vi "ABB Test No Load.vi"() -> ()   [LabVIEW 2017]
uses:
  Temp error msg.ctl
  <vilib>/Analysis/baseanly.llb/Mean (DBL).vi
  ABB global.vi
  <vilib>/Analysis/NI_AALPro.lvlib
  <vilib>/Analysis/NI_AALBase.lvlib
panel:
  in  "Temp error":T1="Error: Temperature measurement "
  in  "Case Constant\n(See Context Help)":i32
  in  "Additional Mech Loss (kW)":dbl
  in  "show fit":bool
  out "Additional Temperatures  (°C)":string[][](table)
  in  "Simulate volts":dbl(slide) max=1800.0
  out "Temperatures  (°C)":string[][](table)
  out "Losses (kW)":string[][](table)
  out "Auto Readings":cluster{"%":dbl[], "Recorded":bool[]}
  out "In Range?":bool[](array[boolean])
  out "saved Readings":dbl[][](array[numeric])
  out "% rated voltage":dbl format="%.1f"
  out "Rated Volts":dbl
  out "Serial number":string
  out "W.O number":string
  out "Power":string[][](table)
  out "Voltage":string[][](table)
  out "Current":string[][](table)
  out "Norma 5000 Error":string
  in  "Record":bool
  out "Readings":string[][](table)
  in  "View":enum16{"Graph", "Readings"}(ring)
  out "Number readings":i32
  out "Status":enum16{"Stopped", "Running"}(ring)
  out "Timedate":string
  in  "End test":bool
  in  "Start":bool
  in  "Read Mode":enum16{"Auto", "Manual"}(ring)
  in  "Exit":bool
  out "Separation of losses":cluster{dbl[], "Best Linear Fit":dbl[]}[](graph)
  # "No Load Test"
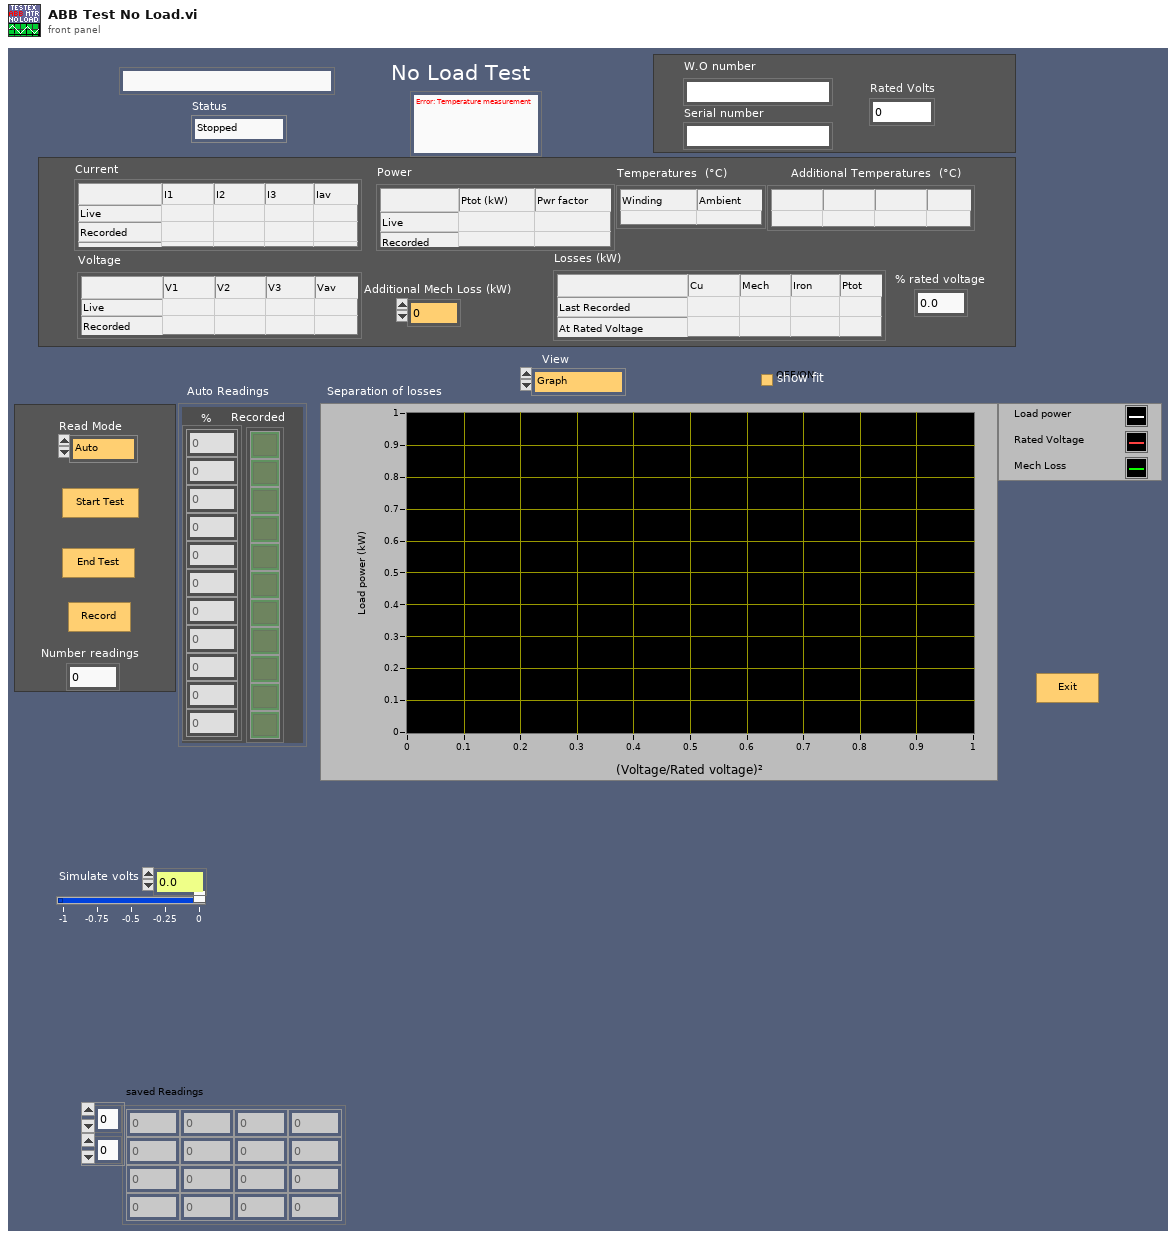
[diagram p1: front panel]
types:
  T1 = typedef "Temp error msg.ctl" = string
  T2 = cluster{"Voltage":dbl, "Current":dbl, "Power":dbl, "power factor":dbl}
  T3 = cluster{"VT Primary":dbl, "VT Secondary":dbl, "CT  Primary":dbl, "CT Secondary":dbl, "Current Shunt":enum16{"Internal", "External"}, "Avg interval":dbl}
  T4 = cluster{"VT Primary":dbl, "VT Secondary":dbl, "CT  Primary":dbl, "CT Secondary":dbl, "Current Shunt":enum16{"Internal", "External"}, "Averaging interval (secs)":dbl}
  T5 = cluster{"Visa sesssion":refnum<visa-resource-name>, "error":errorcluster}
  T6 = cluster{"Simulate Norma":bool, "Norma 5000 Address":u8, "WebDaq IP Address":string, "Simulate cDAQ":bool}
  T7 = cluster{"Number Values":i32, "Tolerance ":dbl, "Value (ratio)":dbl[], "Hold time (sec)":dbl}
  T8 = cluster{"temp. alloc":i32[], "category":i32[], "Category names":string[], "Category none names":string[]}
  T9 = cluster{"PCu":dbl, "Pmech":dbl, "PFe":dbl, "Ptot":dbl, "Ambient":dbl, "I1":dbl, "I2":dbl, "I3":dbl, "Wdg Temp":dbl}
  T10 = cluster{"V":dbl, "A":dbl, "W":dbl, "VA":dbl, "VAr":dbl, "Pf":dbl}
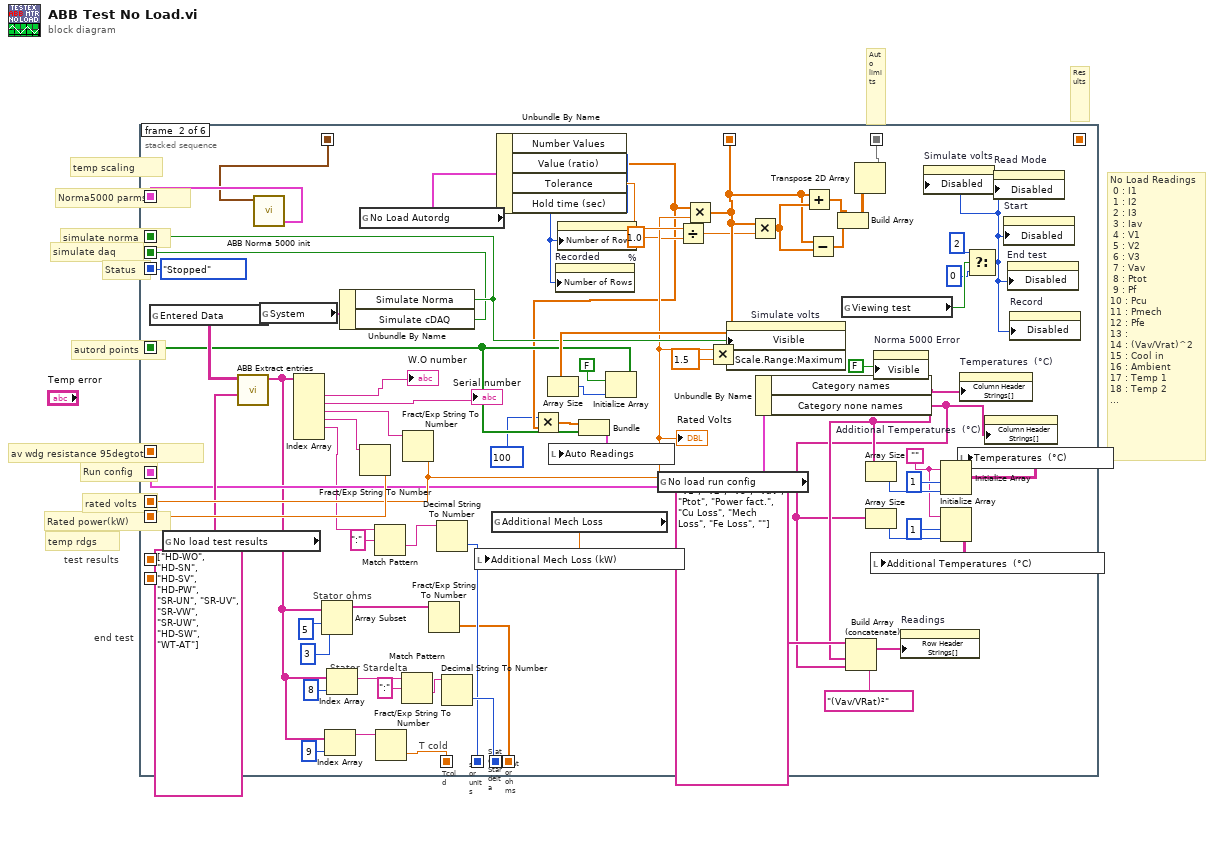
[diagram p0: block diagram]
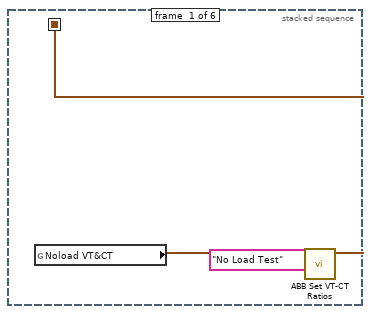
[diagram p2: hidden frame]
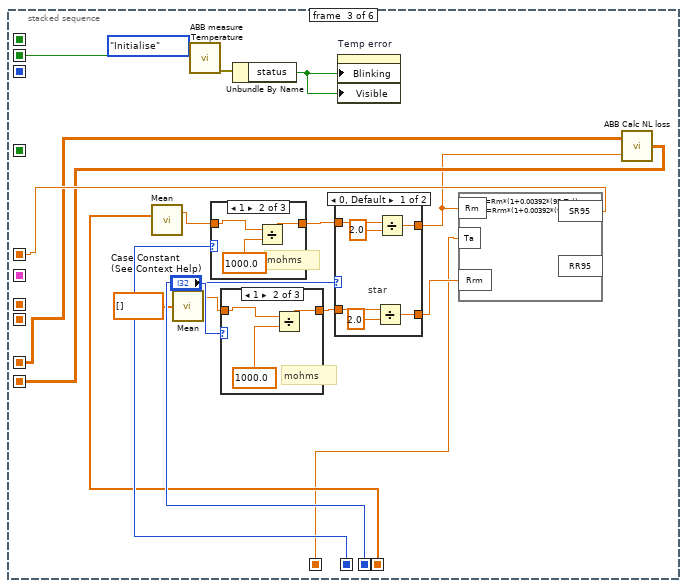
[diagram p3: hidden frame]
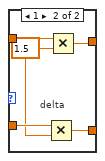
[diagram p4: hidden frame]
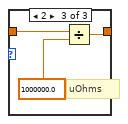
[diagram p6: hidden frame]
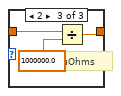
[diagram p8: hidden frame]
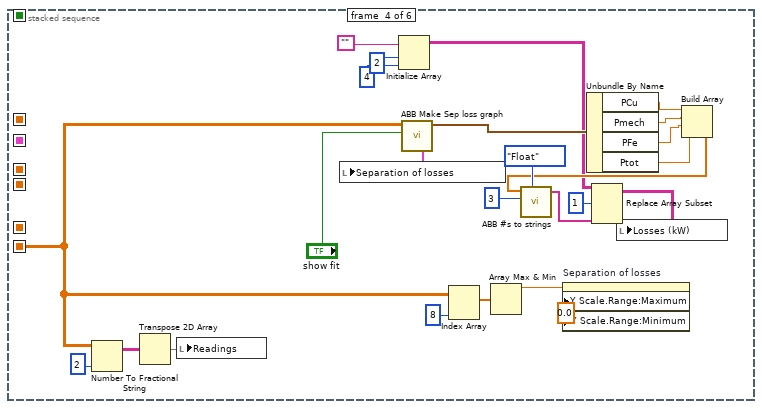
[diagram p9: hidden frame]
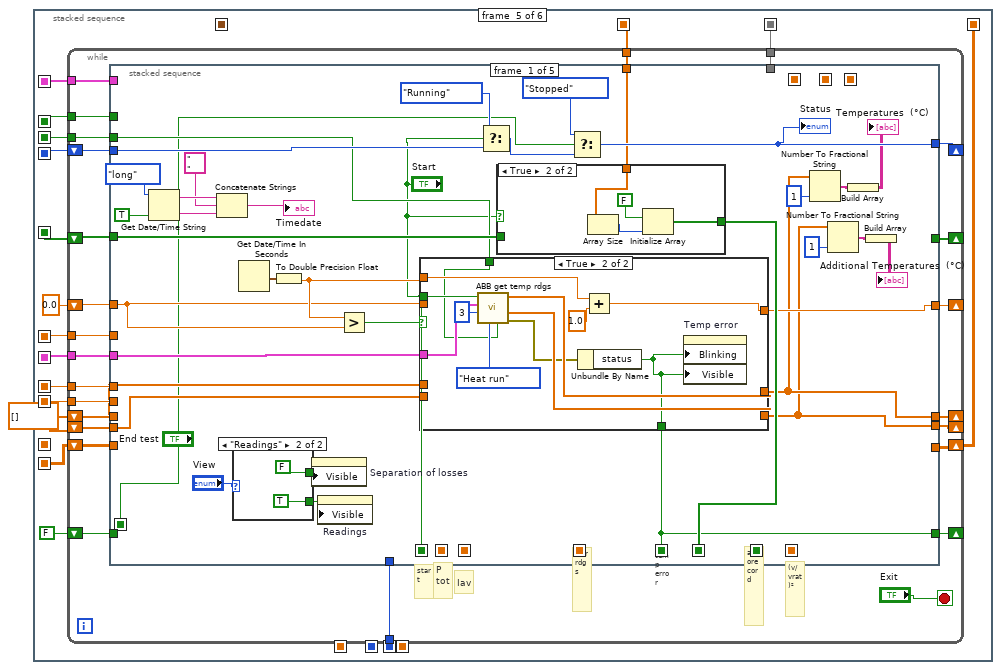
[diagram p10: hidden frame]
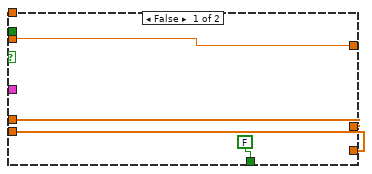
[diagram p11: hidden frame]
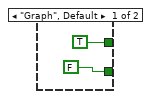
[diagram p13: hidden frame]
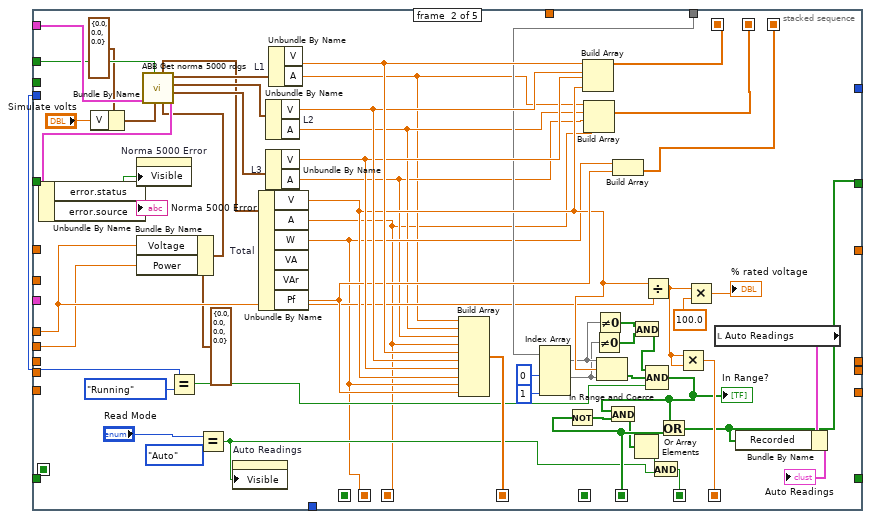
[diagram p14: hidden frame]
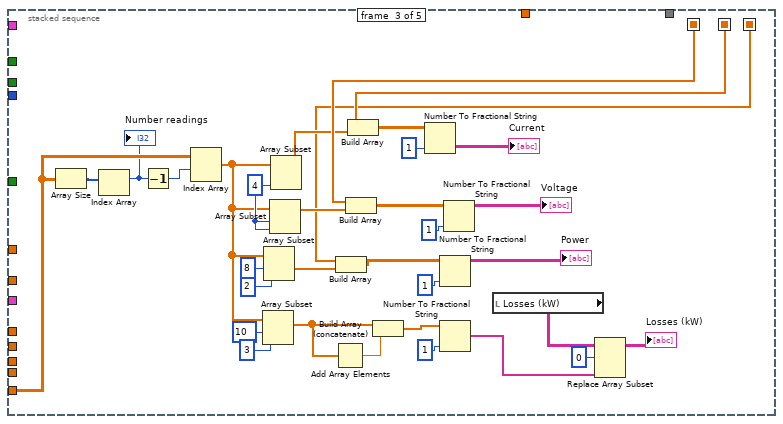
[diagram p15: hidden frame]
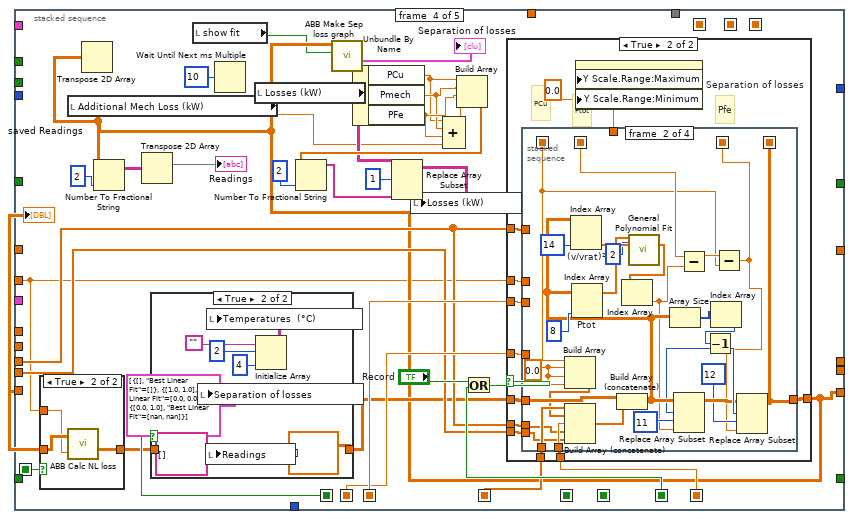
[diagram p16: hidden frame]
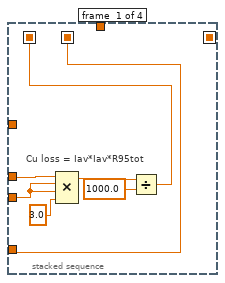
[diagram p20: hidden frame]
diagram:
  # "end test"
  # "test results"
  # "stator ohms"
  # "stator units"
  # "Tcold"
  # "Stator Stardelta"
  # "No Load Readings\n 0 : I1\n 1 : I2\n 2 : I3\n 3 : Iav\n 4 : V1\n 5 : V2\n 6 : V3\n 7 : Vav\n 8 : Ptot\n 9 : Pf\n10 : Pcu\n11 : Pmech\n12 : Pfe\n13 :\n14 : (Vav/Vrat)^2\n15 : Cool in\n16 : Ambient\n17 : Temp 1\n18 : Temp 2\n..."
  # "simulate daq"
  # "temp scaling"
  # "Results"
  # "temp rdgs"
  # "Run config"
  # "Rated power(kW)"
  # "autord points"
  # "Auto limits"
  # "av wdg resistance 95degtot"
  # "rated volts"
  # "simulate norma"
  # "Norma5000 parms"
  # "Status"
  n1 = stacked-sequence {
    seq-local: [_ enum16{"Stopped", "Running"}."Stopped" ("Status") _ _ _ _] -> [_ _ _ _ w160 _]
    seq-local: [_ w73 _ _ _ _] -> [_ _ _ _ w159 w458]
    seq-local: [_ w59 _ _ _ _] -> [_ _ _ _ w158 w457]
    seq-local: [_ w58 _ _ _ _] -> [_ _ _ _ w157 _]
    seq-local: [_ w46 _ _ _ _] -> [_ _ w81 _ _ _]
    seq-local: [_ _ w82 _ _ _] -> [_ _ _ _ w156 _]
    seq-local: [_ w24 _ _ _ _] -> [_ _ _ _ w155 _]
    seq-local: [_ w65 _ _ _ _] -> [_ _ _ _ w153 _]
    seq-local: [_ w63 _ _ _ _] -> [_ _ _ _ w154 _]
    seq-local: [_ w60 _ _ _ _] -> [_ _ _ _ w152 _]
    seq-local: [_ w26 _ _ _ _] -> [_ _ _ _ w150 _]
    seq-local: [_ _ _ _ w149 _] -> [_ _ _ _ _ w455]
    seq-local: [_ w37 _ _ _ _] -> [_ _ w78 _ w148 w452]
    seq-local: [_ w15 _ _ _ _] -> [_ _ w86 _ w146 _]
    seq-local: [w1 _ _ _ _ _] -> [_ w11 _ _ _ w454]
    seq-local: [_ w10 _ _ _ _] -> [_ _ w83 _ _ _]
    seq-local: [_ w9 _ _ _ _] -> [_ _ w87 _ _ _]
    seq-local: [_ w8 _ _ _ _] -> [_ _ w85 _ _ _]
    seq-local: [_ _ w80 _ _ _] -> [_ _ _ w120 w145 _]
    frame #0 {
      n2 = global read "ABB global.vi" "Noload VT&CT"() -> (w3:T3)
      n3 = call "ABB Set VT-CT Ratios.vi"("Test name"="No Load Test", "VT and CT Ratios"=w3) -> ("VT and CT Ratios out"=w1:T4)  [unwired: 9 in]
    }
    frame #1 {
      w28 = ""
      # "T cold"
      # "Stator Stardelta"
      # "Stator ohms"
      n4 = global read "ABB global.vi" "Entered Data"() -> (w55:string[][])
      n5 = global read "ABB global.vi" "No load test results"() -> (w46:dbl[][])
      n6 = call "ABB Extract entries.vi"("Entry IDs"=string[] ["HD-WO", "HD-SN", "HD-SV", "HD-PW", "SR-UN", "SR-UV", "SR-VW", "SR-UW", "HD-SW", "WT-AT"], "Entry table in"=w55) -> ("Selected Entries"=w13:string[])  [unwired: 9 in]
      n7 = call "ABB Norma 5000 init.vi"("VT and CT Ratios"=w11) -> ("norma 5000 parms out"=w73:T5)  [unwired: 10 in]
      n8 = global read "ABB global.vi" "System"() -> (w72:T6)
      n9 = Index Array(array=w13) -> (element #1=→"W.O number":string, element #2=→"Serial number":string, element #3=w52:string, element #4=w51:string, element #5=w6:string)  [unwired: 6 in, 1 out]
      n10 = Array Subset(array=w13, index=5, length=3) -> (w48:string[])
      n11 = Index Array(array=w13, index=9) -> (element=w12:string)
      n12 = Index Array(array=w13, index=8) -> (element=w18:string)
      n13 = Unbundle By Name(w72) -> ("Simulate Norma"=w59:bool, "Simulate cDAQ"=w37:bool)
      n14 = global read "ABB global.vi" "No Load Autordg"() -> (w62:T7)
      n15 = Fract/Exp String To Number(string=w51) -> (number=w60:dbl)  [unwired: 3 in, 1 out]
      n16 = Match Pattern(string=w6, regular expression=":") -> (after substring=w5:string)  [unwired: 1 in, 3 out]
      n17 = Fract/Exp String To Number(string=w12) -> (number=w10:dbl)  [unwired: 3 in, 1 out]
      n18 = Match Pattern(string=w18, regular expression=":") -> (after substring=w16:string)  [unwired: 1 in, 3 out]
      n19 = Fract/Exp String To Number(string=w52) -> (number=w58:dbl)  [unwired: 3 in, 1 out]
      "Rated Volts" <- w58
      n20 = Fract/Exp String To Number(string=w48) -> (number=w8:dbl[])  [unwired: 3 in, 1 out]
      n21 = Decimal String To Number(string=w5) -> (number=w9:i32)  [unwired: 2 in, 1 out]
      n22 = Decimal String To Number(string=w16) -> (number=w15:i32)  [unwired: 2 in, 1 out]
      n23 = global read "ABB global.vi" "Additional Mech Loss"() -> (w4:dbl)
      n24 = local write "Additional Mech Loss (kW)"(w4) -> ()
      n25 = Unbundle By Name(w62) -> ("Number Values"=w25:i32, "Value (ratio)"=w23:dbl[], "Tolerance"=w61:dbl)  [unwired: 1 out]
      n26 = Multiply(x=100 ("Numeric"), y=w23) -> (x*y=w21:dbl[])
      n27 = property on="Recorded" class="Arr (strict)"("Number of Rows"=w25) -> ()  [unwired: 2 in, 2 out]
      n28 = property on="%" class="Arr (strict)"("Number of Rows"=w25) -> ()  [unwired: 2 in, 2 out]
      n29 = global read "ABB global.vi" "No load run config"() -> (w26:T8)
      n30 = Divide(x=w61, y=1.0) -> (x/y=w45:dbl)
      n31 = Multiply(x=w23, y=w58) -> (x*y=w63:dbl[])
      n32 = Array Size(array=w63) -> (size(s)=w70:i32)
      n33 = Initialize Array(FALSE, w70) -> (w24:bool[])
      n34 = Bundle(w21, w24) -> (w22:cluster{dbl[], bool[]})  [unwired: 1 in]
      n35 = local write "Auto Readings"(w22) -> ()
      n36 = Multiply(x=w58, y=1.5) -> (x*y=w56:dbl)
      n37 = property on="Simulate volts" class="Slide (strict)"("Visible"=w59, "Scale.Range:Maximum"=w56) -> ()  [unwired: 2 in, 2 out]
      n38 = Multiply(x=w63, y=w45) -> (x*y=w67:dbl[])
      n39 = Unbundle By Name(w26) -> ("Category names"=w33:string[], "Category none names"=w30:string[])
      n40 = Add(x=w63, y=w67) -> (x+y=w68:dbl[])
      n41 = Subtract(x=w63, y=w67) -> (x-y=w64:dbl[])
      n42 = Build Array(w68, w64) -> (w66:dbl[][])
      n43 = global read "ABB global.vi" "Viewing test"() -> (w41:bool)
      n44 = Build Array (concatenate)(string[] ["I1", "I2", "I3", "Iav", "V1", "V2", "V3", "Vav", "Ptot", "Power fact.", "Cu Loss", "Mech Loss", "Fe Loss", ""], "(Vav/VRat)²", w33, w30) -> (w42:string[])
      n45 = Transpose 2D Array(2D array=w66) -> (transposed array=w65:dbl[][])
      n46 = Array Size(array=w33) -> (size(s)=w35:i32)
      n47 = Array Size(array=w30) -> (size(s)=w27:i32)
      n48 = property on="Norma 5000 Error" class="Str"("Visible"=FALSE) -> ()  [unwired: 2 in, 2 out]
      n49 = property on="Readings" class="Tbl (strict)"("Row Header Strings[]"=w42) -> ()  [unwired: 2 in, 2 out]
      n50 = Initialize Array(w28, 1 ("dimension size"), w35) -> (w32:string[][])
      n51 = Initialize Array(w28, 1 ("dimension size"), w27) -> (w29:string[][])
      n52 = local write "Additional Temperatures  (°C)"(w29) -> ()
      n53 = local write "Temperatures  (°C)"(w32) -> ()
      n54 = property on="Temperatures  (°C)" class="Tbl (strict)"("Column Header Strings[]"=w33) -> ()  [unwired: 2 in, 2 out]
      n55 = Select(t=2, s=w41, f=0) -> (s? t:f=w38:i32)
      n56 = property on="Simulate volts" class="Slide (strict)"("Disabled"=w38) -> ()  [unwired: 2 in, 2 out]
      n57 = property on="Additional Temperatures  (°C)" class="Tbl (strict)"("Column Header Strings[]"=w30) -> ()  [unwired: 2 in, 2 out]
      n58 = property on="Read Mode" class="Enum (strict)"("Disabled"=w38) -> ()  [unwired: 2 in, 2 out]
      n59 = property on="Start" class="Bool"("Disabled"=w38) -> ()  [unwired: 2 in, 2 out]
      n60 = property on="End test" class="Bool"("Disabled"=w38) -> ()  [unwired: 2 in, 2 out]
      n61 = property on="Record" class="Bool"("Disabled"=w38) -> ()  [unwired: 2 in, 2 out]
    }
    frame #2 {
      n62 = call-poly <vilib>:"Mean.vi"("X"=w85) -> ("mean"=w93:dbl)  [unwired: 1 out]
      n63 = call-poly <vilib>:"Mean.vi"("X"=dbl[] []) -> ("mean"=w91:dbl)  [unwired: 1 out]
      n64 = call "ABB measure Temperature.vi"("Simulate"=w78, "Mode"=enum16{"Initialise", "Read", "Close"}."Initialise") -> ("error out"=w76:errorcluster)  [unwired: 7 in, 2 out]
      n65 = case shown="1" w87 {
        tunnel: w93 -> [w112 w115 w118]
        tunnel: [w112 w113 w116] -> w90
        frame 0, Default {
          # "ohms"
        }
        frame 1 {
          # "mohms"
          n66 = Divide(x=w115, y=1000.0) -> (x/y=w113:dbl)
        }
        frame 2 {
          # "uOhms"
          n67 = Divide(x=w118, y=1000000.0) -> (x/y=w116:dbl)
        }
      }
      n68 = case shown="1" "Case Constant\n(See Context Help)" {
        tunnel: w91 -> [w105 w108 w111]
        tunnel: [w105 w106 w109] -> w89
        frame 0, Default {
          # "ohms"
        }
        frame 1 {
          # "mohms"
          n69 = Divide(x=w108, y=1000.0) -> (x/y=w106:dbl)
        }
        frame 2 {
          # "uOhms"
          n70 = Divide(x=w111, y=1000000.0) -> (x/y=w109:dbl)
        }
      }
      n71 = Unbundle By Name(w76) -> ("status"=w75:bool)
      n72 = case shown="0, Default" w86 {
        tunnel: w90 -> [w99 w104]
        tunnel: [w97 w103] -> w79
        tunnel: w89 -> [w96 w102]
        tunnel: [w95 w101] -> w88
        frame 0, Default {
          # "star"
          n73 = Divide(x=w96, y=2.0) -> (x/y=w95:dbl)
          n74 = Divide(x=w99, y=2.0) -> (x/y=w97:dbl)
        }
        frame 1 {
          w100 = 1.5 ("y")
          # "delta"
          n75 = Multiply(x=w102, y=w100) -> (x*y=w101:dbl)
          n76 = Multiply(x=w104, y=w100) -> (x*y=w103:dbl)
        }
      }
      n77 = property on="Temp error" class="Str (strict)"("Blinking"=w75, "Visible"=w75) -> ()  [unwired: 2 in, 2 out]
      n78 = formula code="SR95=Rm*(1+0.00392*(95-Ta));\nRR95=Rrm*(1+0.00392*(95-Ta));"("Rm"=w79, "Ta"=w83, "Rrm"=w88) -> ("SR95"=w82:dbl)  [unwired: 1 out]
      n79 = call "ABB Calc NL loss.vi"("SR95"=w79, "No load test results 2"=w81) -> ("No load test results"=w80:dbl[][])
    }
    frame #3 {
      n80 = Number To Fractional String(number=w120, precision (6)=i16 2) -> (F-format string=w142:string[][])  [unwired: 2 in]
      n81 = Transpose 2D Array(2D array=w142) -> (transposed array=w141:string[][])
      n82 = local write "Readings"(w141) -> ()
      n83 = Initialize Array("", 2, 4) -> (w125:string[][])
      n84 = call "ABB Make Sep loss graph.vi"("Show fit"="show fit", "Results"=w120) -> ("Sep Loss Graph"=w140:cluster{dbl[], dbl[]}[], "Rated V Readings"=w127:T9)  [unwired: 7 in, 1 out]
      n85 = local write "Separation of losses"(w140) -> ()
      n86 = Index Array(array=w120, index (col)=8 ("disabled index (col)")) -> (element=w123:dbl[])  [unwired: 1 in]
      n87 = Array Max & Min(array=w123) -> (max value=w122:dbl)  [unwired: 3 out]
      n88 = property on="Separation of losses" class="XYGraph (strict)"("Y Scale.Range:Maximum"=w122, "Y Scale.Range:Minimum"=0.0) -> ()  [unwired: 2 in, 2 out]
      n89 = Unbundle By Name(w127) -> ("PCu"=w136:dbl, "Pmech"=w135:dbl, "PFe"=w134:dbl, "Ptot"=w133:dbl)
      n90 = Build Array(w136, w135, w134, w133) -> (w126:dbl[])
      n91 = call "ABB #s to strings.vi"("# type"=enum16{"Float", "Relative time HH:MM"}."Float", "Precision"=3, "Numbers in"=w126) -> ("Strings out"=w128:string[])  [unwired: 8 in]
      n92 = Replace Array Subset(array=w125, new element=w128, index (row)=1) -> (w130:string[][])  [unwired: 1 in]
      n93 = local write "Losses (kW)"(w130) -> ()
    }
    frame #4 {
      w147 = dbl[] []
      n94 = while {
        shift-right: [w183] -> _
        shift-left: w160 -> [w184]
        tunnel: w159 -> [w182]
        tunnel: w158 -> [w181]
        tunnel: w157 -> [w180]
        shift-right: [w178] -> w149
        shift-left: w145 -> [w179]
        tunnel: w156 -> [w177]
        shift-right: [w176] -> _
        shift-left: w155 -> [w175]
        tunnel: w154 -> [w174]
        tunnel: w153 -> [w173]
        tunnel: w152 -> [w172]
        shift-right: [w170] -> _
        shift-left: 0.0 -> [w171]
        tunnel: w150 -> [w169]
        shift-right: [w168] -> _
        shift-left: w147 -> [w167]
        tunnel: w148 -> [w166]
        shift-right: [w164] -> _
        shift-left: w147 -> [w165]
        tunnel: w146 -> [w163]
        shift-right: [w162] -> _
        shift-left: FALSE ("status") -> [w161]
        stop <- "Exit" stop-if-true
        # "temp error"
        # "P tot"
        # "Iav"
        # "autorecord"
        # "(v/vrat)²"
        # "pwr rdgs"
        # "start"
        n95 = stacked-sequence {
          seq-local: ["Start" _ _ _ _] -> [_ _ _ w372 _]
          seq-local: [_ w290 _ _ _] -> [_ _ _ w367 _]
          seq-local: [_ w288 _ _ _] -> [_ _ _ w366 _]
          seq-local: [w206 _ _ _ _] -> [_ w283 _ _ _]
          seq-local: [_ w278 _ _ _] -> [_ _ _ w369 _]
          seq-local: [_ w274 _ _ _] -> [_ _ w331 _ _]
          seq-local: [_ w273 _ _ _] -> [_ _ w327 _ _]
          seq-local: [_ w272 _ _ _] -> [_ _ w319 _ _]
          seq-local: [_ w248 _ _ _] -> [_ _ _ w365 _]
          seq-local: [_ w257 _ _ _] -> [_ _ _ w364 _]
          seq-local: ["End test" _ _ _ _] -> [_ _ _ w342 _]
          seq-local: [w186 _ _ _ _] -> [_ _ _ _ w445]
          tunnel: w184 -> [w216 w260 _ _ _]
          tunnel: [w212 _ _ _ _] -> w183
          tunnel: w182 -> [_ w305 _ _ _]
          tunnel: w181 -> [_ w297 _ _ _]
          tunnel: w180 -> [_ w271 _ _ _]
          tunnel: w179 -> [_ _ w337 w343 _]
          tunnel: [_ _ _ w345 _] -> w178
          tunnel: w177 -> [_ _ _ w341 _]
          tunnel: [_ w253 _ _ _] -> w176
          tunnel: w175 -> [w208 _ _ _ _]
          tunnel: w174 -> [w207 _ _ _ _]
          tunnel: w173 -> [_ w286 _ _ _]
          tunnel: w172 -> [_ w255 _ _ _]
          tunnel: w171 -> [w201 _ _ _ _]
          tunnel: [w202 _ _ _ _] -> w170
          tunnel: w169 -> [w200 _ _ _ _]
          tunnel: [w195 _ _ _ _] -> w168
          tunnel: w167 -> [w199 _ _ w363 _]
          tunnel: w166 -> [w198 _ _ _ w442]
          tunnel: w165 -> [w197 _ _ w362 _]
          tunnel: [w189 _ _ _ _] -> w164
          tunnel: w163 -> [_ _ _ _ _]
          tunnel: [w186 _ _ _ _] -> w162
          tunnel: w161 -> [_ _ _ _ w444]
          frame #0 {
            n96 = Get Date/Time String(date format (0)=enum16{"short", "long", "abbreviated"}."long", want seconds? (F)=TRUE) -> (date string=w220:string, time string=w219:string)  [unwired: 1 in]
            n97 = Concatenate Strings(w220, "   ", w219) -> (→"Timedate":string)
            n98 = case shown="\"Readings\"" "View" {
              tunnel: [TRUE FALSE] -> w210
              tunnel: [FALSE TRUE] -> w209
              frame "Graph", Default {
              }
              frame "Readings" {
              }
            }
            n99 = Get Date/Time In Seconds() -> (seconds since 1Jan1904=w204:timestamp)
            n100 = To Double Precision Float(number=w204) -> (double precision float=w203:dbl)
            n101 = property on="Separation of losses" class="XYGraph (strict)"("Visible"=w210) -> ()  [unwired: 2 in, 2 out]
            n102 = property on="Readings" class="Tbl (strict)"("Visible"=w209) -> ()  [unwired: 2 in, 2 out]
            n103 = Greater?(x=w203, y=w201) -> (0:w205:bool)
            n104 = case shown="True" w205 {
              tunnel: w203 -> [_ w238]
              tunnel: [w226 w236] -> w202
              tunnel: w201 -> [w226 _]
              tunnel: w198 -> [_ w229]
              tunnel: w200 -> [_ w235]
              tunnel: [w225 w234] -> w195
              tunnel: w199 -> [w225 _]
              tunnel: w197 -> [w224 _]
              tunnel: [w224 w233] -> w189
              tunnel: "Start" -> [_ w232]
              tunnel: [FALSE ("status") w227] -> w186
              frame False {
              }
              frame True {
                n105 = call "ABB get temp rdgs.vi"("Sim daq"=w229, "sim type"=enum16{"Heat run", "Bearing run"}."Heat run", "# categories"=3, "run config"=w235, "start"=w232) -> ("error out"=w228:errorcluster, "Category none rdgs"=w233:dbl[], "Category rdgs"=w234:dbl[])  [unwired: 3 in, 1 out]
                n106 = Unbundle By Name(w228) -> ("status"=w227:bool)
                n107 = Add(x=w238, y=1.0) -> (x+y=w236:dbl)
                n108 = property on="Temp error" class="Str (strict)"("Blinking"=w227, "Visible"=w227) -> ()  [unwired: 2 in, 2 out]
              }
            }
            n109 = Select(t=enum16{"Stopped", "Running"}."Running", s="Start", f=w216) -> (s? t:f=w214:enum16{"Stopped", "Running"})
            n110 = case shown="True" "Start" {
              tunnel: w207 -> [_ w243]
              tunnel: [w239 w240] -> w206
              tunnel: w208 -> [w239 _]
              frame False {
              }
              frame True {
                n111 = Array Size(array=w243) -> (size(s)=w242:i32)
                n112 = Initialize Array(FALSE, w242) -> (w240:bool[])
              }
            }
            n113 = Select(t=enum16{"Stopped", "Running"}."Stopped", s="End test", f=w214) -> (s? t:f=w212:enum16{"Stopped", "Running"})
            "Status" <- w212
            n114 = Number To Fractional String(number=w195, precision (6)=i16 1) -> (F-format string=w193:string[])  [unwired: 2 in]
            n115 = Number To Fractional String(number=w189, precision (6)=i16 1) -> (F-format string=w191:string[])  [unwired: 2 in]
            n116 = Build Array(w193) -> (→"Temperatures  (°C)":string[][])
            n117 = Build Array(w191) -> (→"Additional Temperatures  (°C)":string[][])
          }
          frame #1 {
            n118 = Bundle By Name(cluster=cluster{"V":dbl, "A":dbl, "pwr factor":dbl} {"V"=0.0, "A"=0.0, "pwr factor"=0.0} ("Simulation rdgs"), "V"="Simulate volts") -> (w267:cluster{"V":dbl, "A":dbl, "pwr factor":dbl})
            n119 = Bundle By Name(cluster=T2 {"Voltage"=0.0, "Current"=0.0, "Power"=0.0, "power factor"=0.0} ("Rated"), "Voltage"=w271, "Power"=w255) -> (w270:T2)
            n120 = call "ABB Get norma 5000 rdgs.vi"("Rated"=w270, "Simulation rdgs"=w267, "simulate"=w297, "norma 5000 parms in"=w305) -> ("norma 5000 parms out"=w299:T5, "L 3"=w300:T10, "L 2"=w301:T10, "L1"=w302:T10, "Total"=w298:T10)  [unwired: 3 in]
            n121 = Unbundle By Name(w299) -> ("error.status"=w304:bool, "error.source"=→"Norma 5000 Error":string)
            n122 = property on="Norma 5000 Error" class="Str"("Visible"=w304) -> ()  [unwired: 2 in, 2 out]
            n123 = Equal?(x=w260, y=enum16{"Stopped", "Running"}."Running") -> (x = y?=w258:bool)
            n124 = Equal?(x="Read Mode", y=enum16{"Auto", "Manual"}."Auto") -> (x = y?=w275:bool)
            n125 = property on="Auto Readings" class="Clust (strict)"("Visible"=w275) -> ()  [unwired: 2 in, 2 out]
            n126 = Unbundle By Name "Total"(w298) -> ("V"=w287:dbl, "A"=w248:dbl, "W"=w257:dbl, "Pf"=w291:dbl)  [unwired: 2 out]
            n127 = Unbundle By Name "L2"(w301) -> ("V"=w293:dbl, "A"=w251:dbl)
            n128 = Unbundle By Name "L3"(w300) -> ("V"=w292:dbl, "A"=w250:dbl)
            n129 = Unbundle By Name "L1"(w302) -> ("V"=w294:dbl, "A"=w249:dbl)
            n130 = Build Array(w249, w251, w250, w248, w294, w293, w292, w287, w257, w291) -> (w290:dbl[])
            n131 = Index Array(array=w286, index (col) #1=0 ("disabled index (col)"), index (col) #2=1 ("index (col)")) -> (element #1=w266:dbl[], element #2=w265:dbl[])  [unwired: 2 in]
            n132 = Not(x=w283) -> (.not. x?=w281:bool[])
            n133 = Build Array(w294, w293, w292, w287) -> (w274:dbl[])
            n134 = Build Array(w249, w251, w250, w248) -> (w273:dbl[])
            n135 = Not Equal To 0?(x=w265) -> (x != 0?=w263:bool[])
            n136 = Not Equal To 0?(x=w266) -> (x != 0?=w264:bool[])
            n137 = In Range and Coerce(upper limit=w266, x=w287, lower limit=w265) -> (In Range?=w282:bool[])  [unwired: 1 out]
            n138 = Build Array(w257, w291) -> (w272:dbl[])
            n139 = And(x=w264, y=w263) -> (x .and. y?=w261:bool[])
            n140 = Divide(x=w287, y=w271) -> (x/y=w289:dbl)
            n141 = Compound Arithmetic op=AND(w261, w282, w258) -> (w262:bool[])
            "In Range?" <- w262
            n142 = And(x=w262, y=w281) -> (x .and. y?=w280:bool[])
            n143 = Or Array Elements(Boolean array=w280) -> (logical OR=w279:bool)
            n144 = And(x=w279, y=w275) -> (x .and. y?=w278:bool)
            n145 = Or(x=w262, y=w283) -> (x .or. y?=w253:bool[])
            n146 = Multiply(x=w289, y=w289) -> (x*y=w288:dbl)
            n147 = Multiply(x=w289, y=100.0) -> (x*y=→"% rated voltage":dbl)
            n148 = local read "Auto Readings"() -> (w254:cluster{"%":dbl[], "Recorded":bool[]})
            n149 = Bundle By Name(cluster=w254, "Recorded"=w253) -> (→"Auto Readings":cluster{"%":dbl[], "Recorded":bool[]})
          }
          frame #2 {
            w334 = 4 ("length")
            n150 = Array Size(array=w337) -> (size(s)=w338:i32[])
            n151 = Index Array(array=w338) -> (element=w313:i32)  [unwired: 1 in]
            "Number readings" <- w313
            n152 = Decrement(x=w313) -> (x-1=w336:i32)
            n153 = Index Array(array=w337, index (row)=w336) -> (element=w316:dbl[])  [unwired: 1 in]
            n154 = Array Subset(array=w316, index=10, length=3) -> (w308:dbl[])
            n155 = Array Subset(array=w316, index=8, length=2) -> (w320:dbl[])
            n156 = Array Subset(array=w316, index=w334, length=w334) -> (w333:dbl[])
            n157 = Array Subset(array=w316, length=w334) -> (w326:dbl[])  [unwired: 1 in]
            n158 = Add Array Elements(numeric array=w308) -> (sum=w306:dbl)
            n159 = Build Array(w319, w320) -> (w321:dbl[][])
            n160 = Build Array(w331, w333) -> (w332:dbl[][])
            n161 = Build Array(w327, w326) -> (w325:dbl[][])
            n162 = Build Array (concatenate)(w308, w306) -> (w307:dbl[])
            n163 = Number To Fractional String(number=w325, precision (6)=i16 1) -> (F-format string=→"Current":string[][])  [unwired: 2 in]
            n164 = Number To Fractional String(number=w321, precision (6)=i16 1) -> (F-format string=→"Power":string[][])  [unwired: 2 in]
            n165 = Number To Fractional String(number=w307, precision (6)=i16 1) -> (F-format string=w309:string[])  [unwired: 2 in]
            n166 = Number To Fractional String(number=w332, precision (6)=i16 1) -> (F-format string=→"Voltage":string[][])  [unwired: 2 in]
            n167 = local read "Losses (kW)"() -> (w312:string[][])
            n168 = Replace Array Subset(array=w312, new element=w309, index (row)=0) -> (→"Losses (kW)":string[][])  [unwired: 1 in]
          }
          frame #3 {
            n169 = case shown="True" w342 {
              tunnel: [w373 w375] -> w344
              tunnel: w343 -> [w373 w376]
              tunnel: w341 -> [_ w374]
              frame False {
              }
              frame True {
                n170 = call "ABB Calc NL loss.vi"("SR95"=w374, "No load test results 2"=w376) -> ("No load test results"=w375:dbl[][])
              }
            }
            n171 = local read "Additional Mech Loss (kW)"() -> (w339:dbl)
            n172 = case shown="True" w372 {
              tunnel: w344 -> [w377 _]
              tunnel: [w377 dbl[][] []] -> w361
              frame False {
              }
              frame True {
                n173 = local write "Separation of losses"(cluster{dbl[], "Best Linear Fit":dbl[]}[] [{[], "Best Linear Fit"=[]}, {[1.0, 1.0], "Best Linear Fit"=[0.0, 0.0]}, {[0.0, 1.0], "Best Linear Fit"=[nan, nan]}] ("Separation of losses")) -> ()
                n174 = local write "Readings"(string[][] [] ("Readings")) -> ()
                n175 = Initialize Array("", 2 ("dimension size"), 4 ("dimension size")) -> (w378:string[][])
                n176 = local write "Temperatures  (°C)"(w378) -> ()
              }
            }
            n177 = local read "show fit"() -> (w340:bool)
            n178 = Wait Until Next ms Multiple(millisecond multiple=u32 10) -> ()  [unwired: 1 out]
            n179 = local read "Losses (kW)"() -> (w351:string[][])
            n180 = Or(x="Record", y=w369) -> (x .or. y?=w370:bool)
            n181 = case shown="True" w370 {
              tunnel: w361 -> [w385 w397]
              tunnel: [w385 w396] -> w345
              tunnel: w367 -> [_ w395]
              tunnel: w363 -> [_ w394]
              tunnel: w366 -> [_ w393]
              tunnel: w341 -> [_ w392]
              tunnel: w365 -> [_ w391]
              tunnel: w363 -> [_ w390]
              tunnel: w364 -> [_ w389]
              tunnel: w362 -> [_ w386]
              frame False {
              }
              frame True {
                # "Pfe"
                # "Ptot"
                # "PCu"
                n182 = stacked-sequence {
                  seq-local: [w401 _ _ _] -> [_ w409 _ _]
                  seq-local: [w399 _ _ _] -> [_ w423 _ _]
                  seq-local: [_ w411 _ _] -> [_ _ _ _]
                  seq-local: [_ w415 _ _] -> [_ _ w439 _]
                  tunnel: w397 -> [_ w431 _ _]
                  tunnel: [_ w415 _ _] -> w396
                  tunnel: w395 -> [_ w429 _ _]
                  tunnel: w394 -> [_ w413 w433 _]
                  tunnel: w393 -> [_ w414 _ _]
                  tunnel: w392 -> [w404 _ _ _]
                  tunnel: w391 -> [w403 _ _ _]
                  tunnel: w390 -> [_ _ _ _]
                  tunnel: w389 -> [w399 _ _ _]
                  tunnel: [_ _ w438 _] -> w387
                  tunnel: w386 -> [_ w412 _ _]
                  frame #0 {
                    # "Cu loss = Iav*Iav*R95tot"
                    n183 = Compound Arithmetic op=MULTIPLY(w404, w403, w403, 3.0 ("value")) -> (w402:dbl)
                    n184 = Divide(x=w402, y=1000.0) -> (x/y=w401:dbl)
                  }
                  frame #1 {
                    w408 = 0.0 ("element")
                    n185 = Build Array(w409, w408, w408, w408) -> (w427:dbl[])
                    n186 = Build Array (concatenate)(w429, w427, w414, w413, w412) -> (w430:dbl[])
                    n187 = Build Array (concatenate)(w431, w430) -> (w422:dbl[][])
                    n188 = Index Array "(v/vrat)²"(array=w422, index (col)=14 ("disabled index (col)")) -> (element=w424:dbl[])  [unwired: 1 in]
                    n189 = Index Array "Ptot"(array=w422, index (col)=8 ("disabled index (col)")) -> (element=w425:dbl[])  [unwired: 1 in]
                    n190 = call <vilib>:"General Polynomial Fit.vi"("Y"=w425, "polynomial order"=2, "X"=w424) -> ("Polynomial Coefficients"=w406:dbl[])  [unwired: 9 in, 3 out]
                    n191 = Index Array(array=w406) -> (element=w405:dbl)  [unwired: 1 in]
                    n192 = Array Size(array=w422) -> (size(s)=w421:i32[])
                    n193 = Subtract(x=w423, y=w405) -> (x-y=w410:dbl)
                    n194 = Index Array(array=w421) -> (element=w420:i32)  [unwired: 1 in]
                    n195 = Decrement(x=w420) -> (x-1=w419:i32)
                    n196 = Replace Array Subset(array=w422, new element=w405, index (row)=w419, index (col)=11) -> (w418:dbl[][])
                    n197 = Subtract(x=w410, y=w409) -> (x-y=w411:dbl)
                    n198 = Replace Array Subset(array=w418, new element=w411, index (row)=w419, index (col)=12) -> (w415:dbl[][])
                  }
                  frame #2 {
                    n199 = Index Array(array=w439, index (col)=8 ("disabled index (col)")) -> (element=w440:dbl[])  [unwired: 1 in]
                    n200 = Number To Fractional String(number=w433, precision (6)=i16 1) -> (F-format string=w434:string[])  [unwired: 2 in]
                    n201 = Array Max & Min(array=w440) -> (max value=w438:dbl)  [unwired: 3 out]
                    n202 = local read "Temperatures  (°C)"() -> (w437:string[][])
                    n203 = Replace Array Subset(array=w437, new element=w434, index (row)=1) -> (w436:string[][])  [unwired: 1 in]
                    n204 = local write "Temperatures  (°C)"(w436) -> ()
                  }
                  frame #3 {
                  }
                }
                n205 = property on="Separation of losses" class="XYGraph (strict)"("Y Scale.Range:Maximum"=w387, "Y Scale.Range:Minimum"=0.0) -> ()  [unwired: 2 in, 2 out]
              }
            }
            n206 = Transpose 2D Array(2D array=w345) -> ()  [unwired: 1 out]
            n207 = Number To Fractional String(number=w345, precision (6)=i16 2) -> (F-format string=w348:string[][])  [unwired: 2 in]
            n208 = Transpose 2D Array(2D array=w348) -> (transposed array=→"Readings":string[][])
            n209 = call "ABB Make Sep loss graph.vi"("Show fit"=w340, "Results"=w345) -> ("Sep Loss Graph"=→"Separation of losses":cluster{dbl[], dbl[]}[], "Rated V Readings"=w350:T9)  [unwired: 7 in, 1 out]
            n210 = Unbundle By Name(w350) -> ("PCu"=w355:dbl, "Pmech"=w356:dbl, "PFe"=w357:dbl)
            n211 = Compound Arithmetic op=ADD(w355, w356, w357, w339) -> (w358:dbl)
            n212 = Build Array(w355, w356, w357, w358) -> (w359:dbl[])
            n213 = Number To Fractional String(number=w359, precision (6)=2 ("Precision")) -> (F-format string=w354:string[])  [unwired: 2 in]
            n214 = Replace Array Subset(array=w351, new element=w354, index (row)=1) -> (w352:string[][])  [unwired: 1 in]
            n215 = local write "Losses (kW)"(w352) -> ()
            "saved Readings" <- w343
          }
          frame #4 {
            n216 = Not(x=w444) -> (.not. x?=w443:bool)
            n217 = And(x=w443, y=w445) -> (x .and. y?=w446:bool)
            n218 = case shown="True" w446 {
              tunnel: w442 -> [_ w447]
              frame False {
              }
              frame True {
                # "Reset CDAQ after temp error"
                n219 = stacked-sequence {
                  tunnel: w447 -> [w448 w450]
                  frame #0 {
                    n220 = call "ABB measure Temperature.vi"("Simulate"=w448, "Mode"=enum16{"Initialise", "Read", "Close"}."Close") -> ()  [unwired: 7 in, 3 out]
                  }
                  frame #1 {
                    n221 = call "ABB measure Temperature.vi"("Simulate"=w450, "Mode"=enum16{"Initialise", "Read", "Close"}."Initialise") -> ()  [unwired: 7 in, 3 out]
                  }
                }
              }
            }
          }
        }
      }
    }
    frame #5 {
      n222 = case shown="False" w457 {
        tunnel: w458 -> [w476 _]
        frame False {
          n223 = Unbundle By Name(w476) -> ("Visa sesssion"=w475:refnum<visa-resource-name>, "error"=w474:errorcluster)
          n224 = call "LNOPA01 Error Query.vi"("error in (no error)"=w474, "VISA session"=w475) -> ("error out"=w477:errorcluster, "dup VISA session"=w478:refnum<visa-resource-name>)  [unwired: 6 in, 2 out]
          n225 = call "LNOPA01 Close.vi"("error in (no error)"=w477, "VISA session"=w478) -> ("error out"=w479:errorcluster)  [unwired: 9 in]
          n226 = call <vilib>:"Simple Error Handler.vi"("error in (no error)"=w479) -> ()  [unwired: 4 in, 5 out]
        }
        frame True {
        }
      }
      n227 = call "ABB measure Temperature.vi"("Simulate"=w452, "Mode"=enum16{"Initialise", "Read", "Close"}."Close") -> ()  [unwired: 7 in, 3 out]
      n228 = global read "ABB global.vi" "Viewing test"() -> (w456:bool)
      n229 = case shown="False" w456 {
        tunnel: w455 -> [w463 _]
        tunnel: w454 -> [w459 _]
        frame False {
          n230 = global read "ABB global.vi" "Current test"() -> (w462:path)
          n231 = Two Button Dialog(message="Save results?", 1:"Discard" ("F button name (\"Cancel\")"), 2:"Save" ("T button name (\"OK\")")) -> (T button?=w464:bool)
          n232 = case shown="True" w464 {
            tunnel: w463 -> [_ w468]
            tunnel: w462 -> [_ w467]
            tunnel: w459 -> [_ w466]
            frame False {
            }
            frame True {
              n233 = stacked-sequence {
                tunnel: w468 -> [w471 _]
                tunnel: w467 -> [_ w472]
                tunnel: w466 -> [w470 _]
                frame #0 {
                  n234 = global write "ABB global.vi" "No load test results"(w471) -> ()
                  n235 = global write "ABB global.vi" "Noload VT&CT"(w470) -> ()
                  n236 = global write "ABB global.vi" "Additional Mech Loss"("Additional Mech Loss (kW)") -> ()
                }
                frame #1 {
                  n237 = call "ABB Load-Save results.vi"("Path"=w472, "Mode"=enum16{"LOAD", "Save"}."Save") -> ()  [unwired: 10 in]
                }
              }
            }
          }
        }
        frame True {
        }
      }
    }
  }
